vi "Run1TonWithoutWaveformDig.vi"() -> ()   [LabVIEW 2014]
doc: "Use this template to build a producer/consumer design pattern with events to produce queue items. Use this design pattern instead of the User Interface Event Handler pattern for user interfaces when you want to execute code asynchronously in response to an event without slowing the user interface responsiveness."
uses:
  <vilib>/addons/h5labview2/base/hid_t.ctl
  DatasetNames.ctl
  Program Files (x86)/CAEN/Comm/labview/CAENComm.lvlib
panel:
  out "Time Data (E-4 s)":T1
  in  "Monitoring Delay (ms)":u16=100 caption="Monitoring Delay (ms) (TDC, QDC, Dig, Time)"
  out "Duty Factor":dbl(graph)
  in  "?":T2(tab)
  out "TDC Histograms":u16[][](graph)
  out "QDC Histograms":u16[][](graph)
  out "Scaler Rates":T3(graph)
  in  "Scaler Delay (s)":sgl=10.0
  out "Time Histogram":u16[][](graph)
  in  "Max Hist Time (s)":sgl=0.25 format="%#_13g"
  in  "Time # Bins":i32=1000
  out "Temp Chart":dynamicdata(graph)
  out "Total Samples":sgl caption="Number of Samples Being Averaged"
  out "Mean":sgl
  in  "Temp Delay (s)":sgl=1.0
  in  "Max Samples":u32=600
  out "# elements in queue":i32
  out "Acquiring?":bool
  out "Scaler Data":u32[](array[numeric])
  out "Acquisition\nErrors":errorcluster
  in  "Clear Acquisition Errors":bool
  in  "QDC threshold":u16=1
  in  "Start Acquisition":bool
  out "# Events Written":i32
  in  "# Events to\nRecord":i32
  out "Analysis\nErrors":errorcluster
  in  "Calibrate Verniers":bool
  in  "Stop Acquisition":bool
  in  "Configure Output":bool
  in  "Calibrate Pedestals":bool
  in  "stop":bool
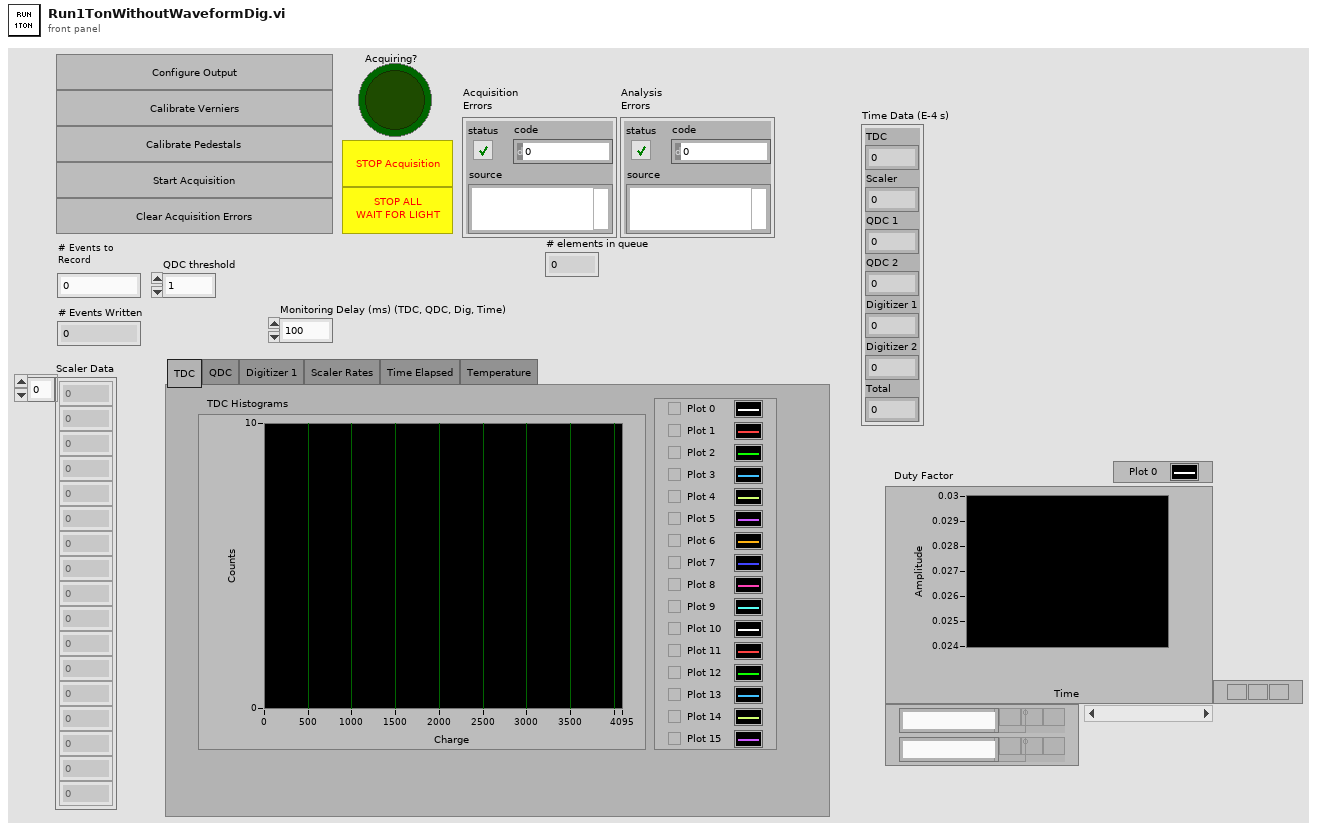
[diagram p1: front panel]
types:
  T1 = cluster{"TDC":u16, "Scaler":u16, "QDC 1":u16, "QDC 2":u16, "Digitizer 1":u16, "Digitizer 2":u16, "Total":u16}
  T2 = enum32{"TDC", "QDC", "Digitizer 1", "Scaler Rates", "Time Elapsed", "Temperature"}
  T3 = cluster{"[0]":dbl, "[1]":dbl, "[2]":dbl, "[3]":dbl}
  T4 = typedef "hid_t.ctl" = i32
  T5 = cluster{"State":enum16{"Startup", "Initialise", "Event OK", "Discard Event", "Exit", "Close"}, "Data":variant}
  T6 = typedef "DatasetNames.ctl" = enum16{"TDC", "Scaler", "QDC_1", "QDC_2", "Digitizer_1", "Digitizer_2", "Event_Time", "Event_Temp"}
  T7 = cluster{"TDC Data":u32[], "Scaler Data":u32[], "QDC 1 Data":u32[], "QDC 2 Data":u32[], "Event Start UNIX Time":dbl}
  T8 = enum16{"Startup", "Initialise", "Event OK", "Discard Event", "Exit", "Close"}
  T9 = cluster{"[0]":dbl, "[1]":dbl, "[2]":dbl, "[3]":dbl}[]
  T10 = cluster{"Channel":u8, "QDC Data":u16, "LowRange?":bool}[]
  T11 = cluster{"Data out[0]":u16, "Data out[1]":u16, "Data out[2]":u16, "Data out[3]":u16, "Data out[4]":u16, "Data out[5]":u16, "Data out[6]":u16}
  T12 = enum16{"Configure", "Initialise", "Run", "Close"}
  T13 = cluster{"TDC":u32, "Scaler":u32, "QDC 1":u32, "QDC 2":u32, "Digitizer 1":u32, "Digitizer 2":u32}
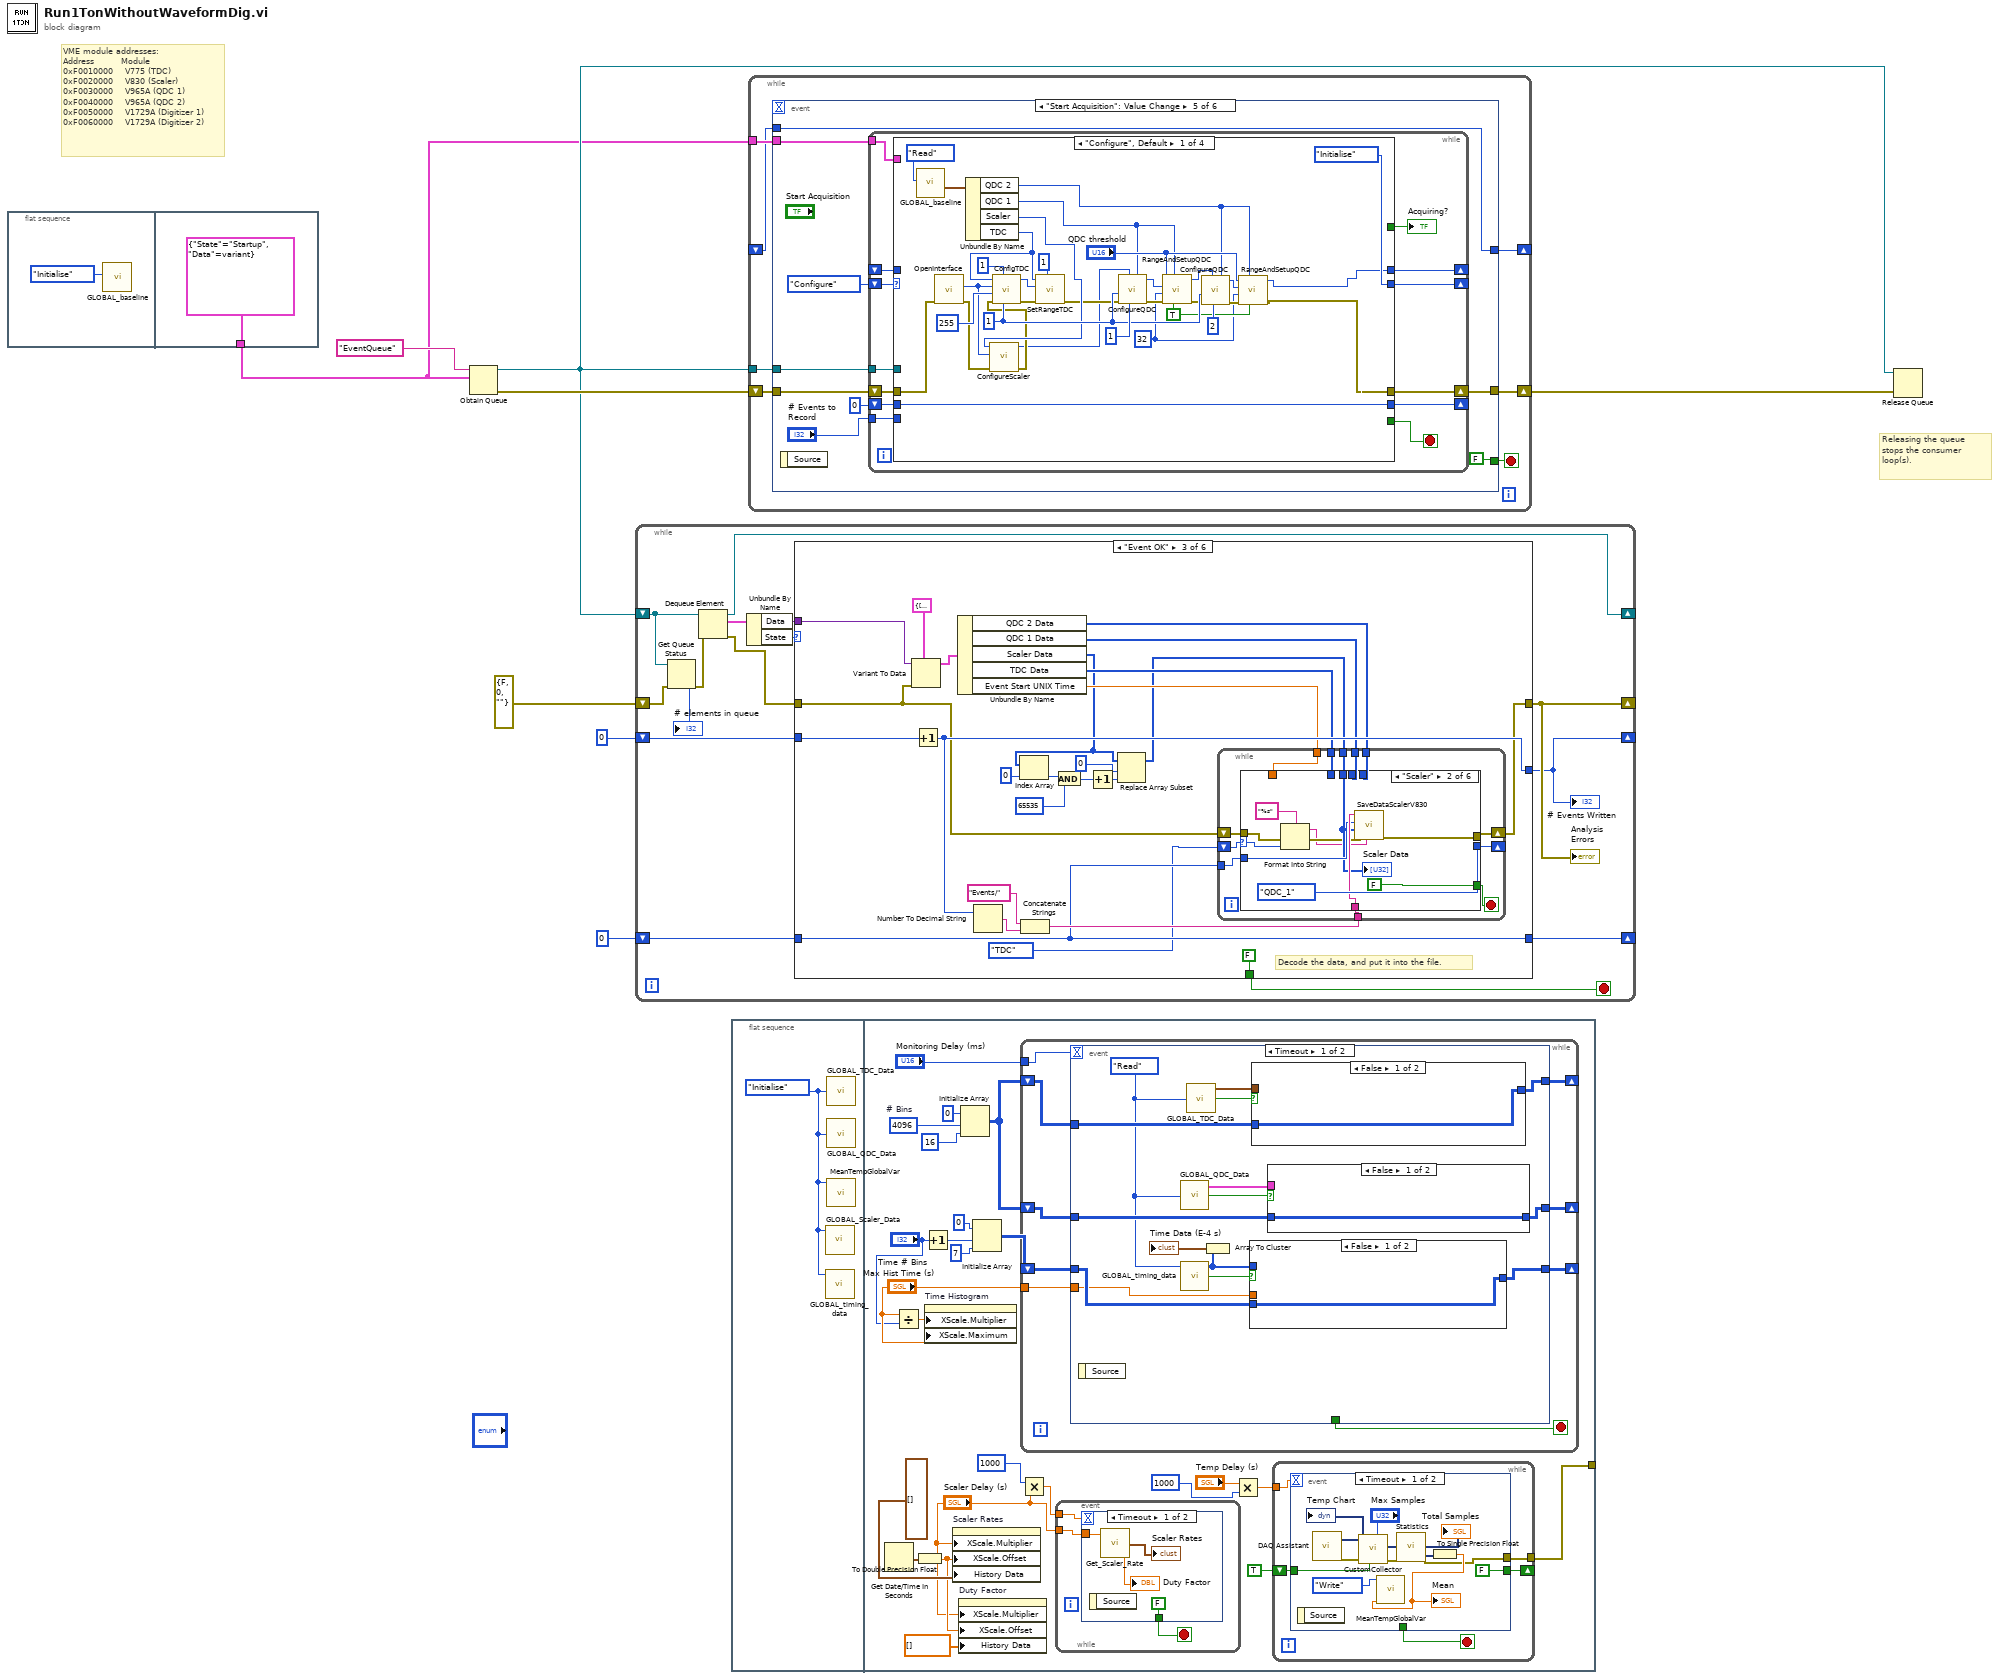
[diagram p0: block diagram]
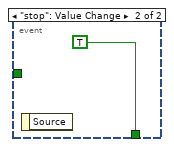
[diagram p2: hidden frame]
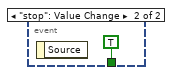
[diagram p3: hidden frame]
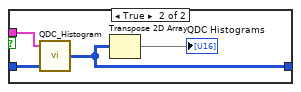
[diagram p4: hidden frame]
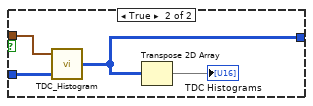
[diagram p5: hidden frame]
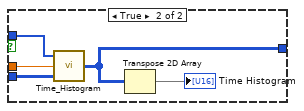
[diagram p6: hidden frame]
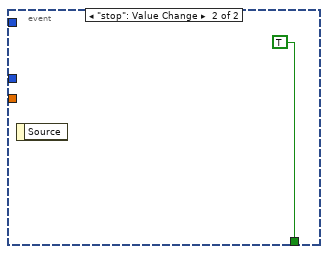
[diagram p7: hidden frame]
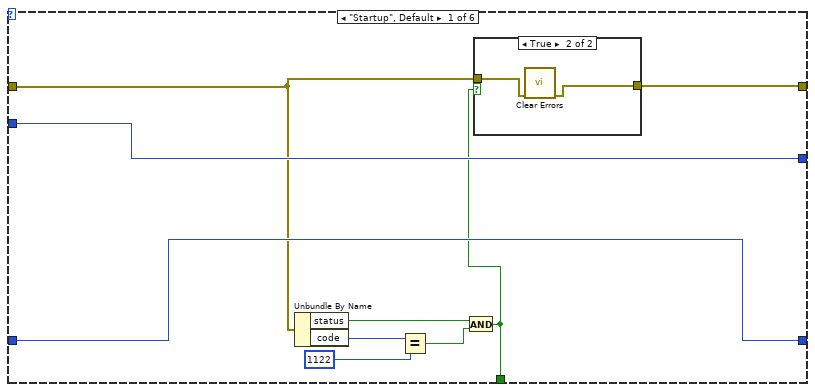
[diagram p8: hidden frame]
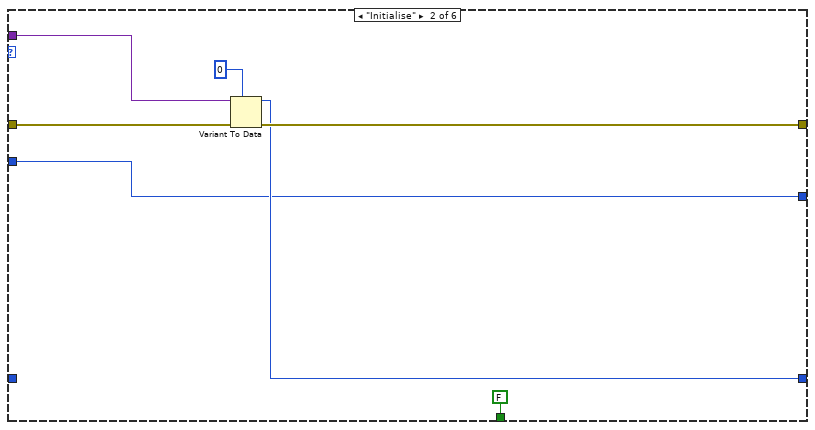
[diagram p10: hidden frame]
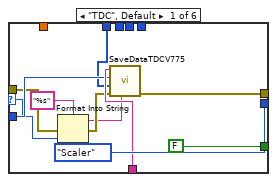
[diagram p11: hidden frame]
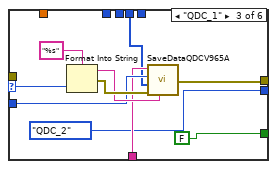
[diagram p12: hidden frame]
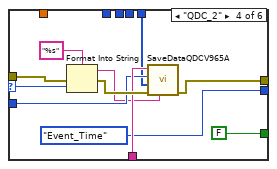
[diagram p13: hidden frame]
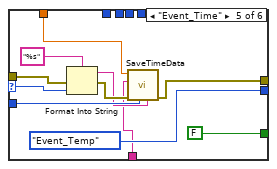
[diagram p14: hidden frame]
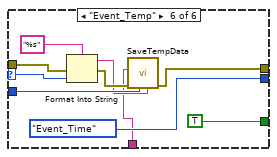
[diagram p15: hidden frame]
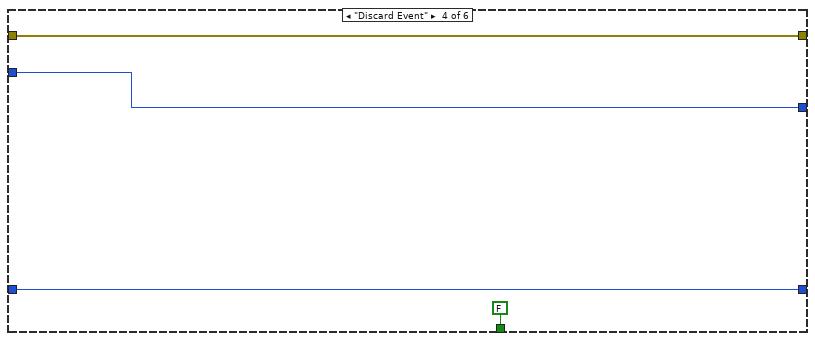
[diagram p16: hidden frame]
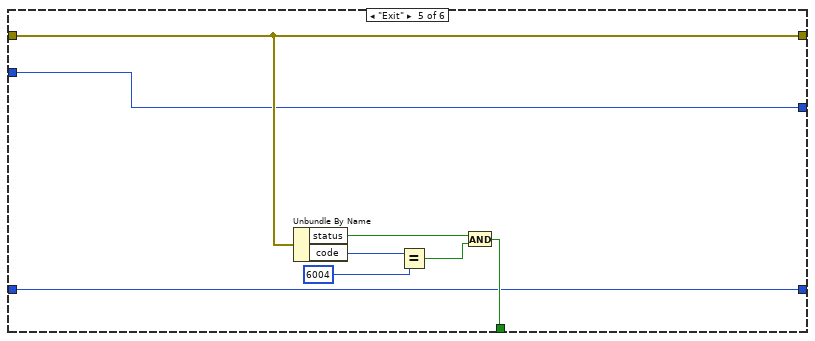
[diagram p17: hidden frame]
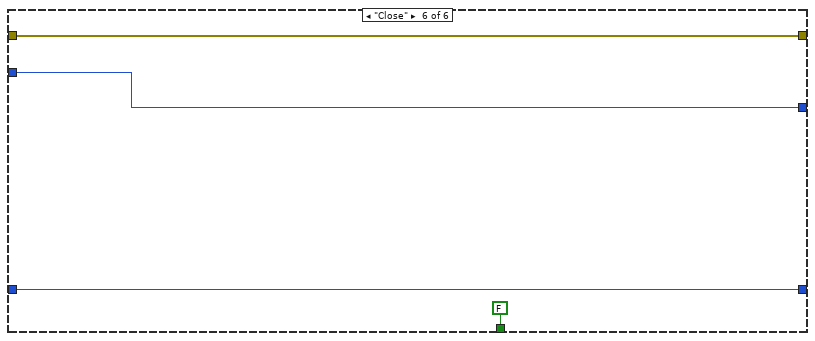
[diagram p18: hidden frame]
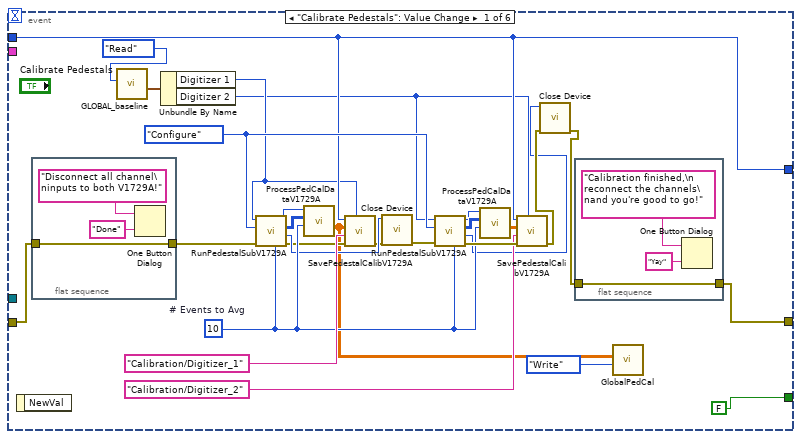
[diagram p19: hidden frame]
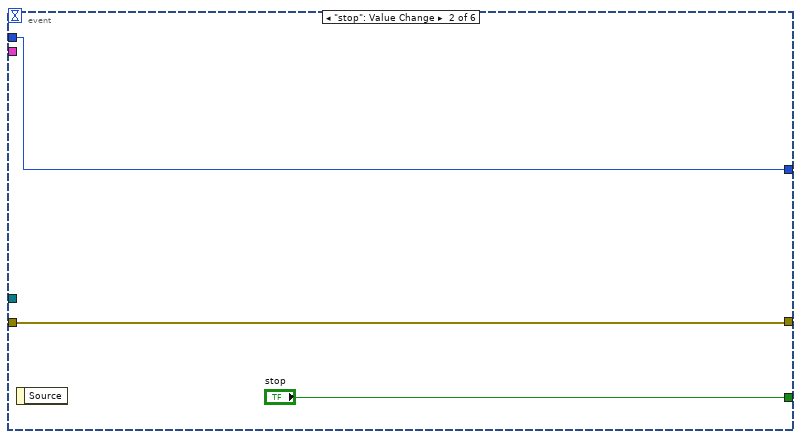
[diagram p20: hidden frame]
diagram:
  # "VME module addresses:\nAddress         Module\n0xF0010000    V775 (TDC)\n0xF0020000    V830 (Scaler)\n0xF0030000    V965A (QDC 1)\n0xF0040000    V965A (QDC 2)\n0xF0050000    V1729A (Digitizer 1)\n0xF0060000    V1729A (Digitizer 2)"
  # "Releasing the queue stops the consumer loop(s)."
  n1 = flat-sequence {
    tunnel: [T5 {"State"=enum."Startup", "Data"=variant}] -> w1
    frame #0 {
      n2 = call "GLOBAL_baseline.vi"("State"=enum16{"Initialise", "Write", "Read"}."Initialise") -> ()  [unwired: 10 in, 1 out]
    }
    frame #1 {
    }
  }
  n3 = Obtain Queue(name (unnamed)="EventQueue", element data type=w1) -> (queue out=w3:refnum<queue>, error out=w8:errorcluster)  [unwired: 3 in, 1 out]
  n4 = while {
    shift-right: [w16] -> _
    shift-left: errorcluster {"status"=FALSE, "code"=0, "source"=""} ("error out") -> [w14]
    shift-right: [w21] -> _
    shift-left: w3 -> [w12]
    shift-right: [w19] -> _
    shift-left: T4 0 ("File Handle") -> [w18]
    shift-right: [w15] -> _
    shift-left: 0 -> [w17]
    stop <- w20 stop-if-true
    n5 = Get Queue Status(queue=w12, error in (no error)=w14) -> (error out=w13:errorcluster, # elements in queue=→"# elements in queue":i32)  [unwired: 1 in, 6 out]
    n6 = Dequeue Element(queue=w12, error in (no error)=w13) -> (queue out=w21:refnum<queue>, element=w25:T5, error out=w22:errorcluster)  [unwired: 1 in, 1 out]
    n7 = Unbundle By Name(w25) -> ("Data"=w23:variant, "State"=w24:T8)
    n8 = case shown="\"Event OK\"" w24 {
      tunnel: w23 -> [_ w42 w68 _ _ _]
      tunnel: w22 -> [w28 w41 w57 w149 w152 w161]
      tunnel: [w26 w40 w55 w149 w152 w161] -> w16
      tunnel: [w27 FALSE FALSE FALSE w153 FALSE] -> w20
      tunnel: [w30 w39 w60 w147 w151 w159] -> w19
      tunnel: w18 -> [w30 _ w60 w147 w151 w159]
      tunnel: w17 -> [w29 w38 w67 w146 w150 w158]
      tunnel: [w29 w38 w66 w146 w150 w158] -> w15
      frame "Startup", Default {
        n9 = Unbundle By Name(w28) -> ("status"=w34:bool, "code"=w32:i32)
        n10 = Equal?(x=w32, y=1122) -> (x = y?=w33:bool)
        n11 = And(x=w34, y=w33) -> (x .and. y?=w27:bool)
        n12 = case shown="True" w27 {
          tunnel: w28 -> [w35 w37]
          tunnel: [w35 w36] -> w26
          frame False {
          }
          frame True {
            n13 = call <vilib>:"Clear Errors.vi"("error in (no error)"=w37) -> ("error out"=w36:errorcluster)  [unwired: 5 in, 1 out]
          }
        }
      }
      frame "Initialise" {
        n14 = Variant To Data(error in=w41, type=T4 0 ("File Handle"), Variant=w42) -> (data=w39:T4, error out=w40:errorcluster)
      }
      frame "Event OK" {
        # "Decode the data, and put it into the file."
        n15 = Variant To Data(error in=w57, type=T7 {"TDC Data"=[], "Scaler Data"=[], "QDC 1 Data"=[], "QDC 2 Data"=[], "Event Start UNIX Time"=0.0}, Variant=w68) -> (data=w62:T7)  [unwired: 1 out]
        n16 = Increment(x=w67) -> (x+1=w66:i32)
        n17 = Unbundle By Name(w62) -> ("QDC 2 Data"=w59:u32[], "QDC 1 Data"=w58:u32[], "Scaler Data"=w49:u32[], "TDC Data"=w56:u32[], "Event Start UNIX Time"=w53:dbl)
        n18 = Number To Decimal String(number=w66) -> (decimal integer string=w64:string)  [unwired: 1 in]
        n19 = Index Array(array=w49, index=0) -> (element=w51:u32)
        n20 = Concatenate Strings("Events/", w64) -> (w61:string)
        n21 = And(x=w51, y=u32 65535) -> (x .and. y?=w48:u32)
        n22 = Increment(x=w48) -> (x+1=w45:u32)
        n23 = Replace Array Subset(array=w49, new element=w45, index=0) -> (w46:u32[])
        n24 = while {
          tunnel: w61 -> [w81]
          tunnel: w60 -> [w80]
          tunnel: w59 -> [w78]
          tunnel: w58 -> [w77]
          shift-right: [w74] -> w55
          shift-left: w57 -> [w79]
          tunnel: w46 -> [w76]
          tunnel: w56 -> [w75]
          shift-right: [w73] -> _
          shift-left: DatasetNames."TDC" -> [w72]
          tunnel: w53 -> [w70]
          stop <- w71 stop-if-true
          n25 = case shown="\"Scaler\"" w72 {
            selector: w72 -> [w82 w96 w110 w123 w134 w144]
            tunnel: [w90 w101 w107 w116 w128 w138] -> w74
            tunnel: w80 -> [w88 w99 w109 w119 w129 w139]
            tunnel: w81 -> [w89 w100 w108 w120 w126 w136]
            tunnel: w79 -> [w85 w95 _ w122 w131 w141]
            tunnel: w78 -> [_ _ _ w118 _ _]
            tunnel: w77 -> [_ _ w106 _ _ _]
            tunnel: [DatasetNames."Scaler" DatasetNames."QDC_1" DatasetNames."QDC_2" DatasetNames."Event_Time" DatasetNames."Event_Temp" DatasetNames."Event_Time"] -> w73
            tunnel: [FALSE FALSE FALSE FALSE FALSE TRUE] -> w71
            tunnel: w76 -> [_ w98 _ _ _ _]
            tunnel: w75 -> [w87 _ _ _ _ _]
            tunnel: w70 -> [_ _ _ _ w125 _]
            frame "TDC", Default {
              n26 = Format Into String(format string="%s", error in=w85, w82) -> (resulting string=w83:string, error out=w84:errorcluster)  [unwired: 1 in]
              n27 = call "SaveDataTDCV775.vi"("Module"=w83, "error in (no error)"=w84, "Buff"=w87, "File Handle"=w88, "String"=w89) -> ("error out"=w90:errorcluster)  [unwired: 5 in, 1 out]
            }
            frame "Scaler" {
              n28 = Format Into String(format string="%s", error in=w95, w96) -> (resulting string=w93:string, error out=w94:errorcluster)  [unwired: 1 in]
              n29 = call "SaveDataScalerV830.vi"("Module"=w93, "error in (no error)"=w94, "Buff"=w98, "File Handle"=w99, "Group Name"=w100) -> ("error out"=w101:errorcluster)  [unwired: 6 in]
              "Scaler Data" <- w98
            }
            frame "QDC_1" {
              n30 = Format Into String(format string="%s", w110) -> (resulting string=w111:string, error out=w112:errorcluster)  [unwired: 2 in]
              n31 = call "SaveDataQDCV965A.vi"("Module"=w111, "error in (no error)"=w112, "Buff"=w106, "File Handle"=w109, "String"=w108) -> ("error out"=w107:errorcluster)  [unwired: 5 in, 1 out]
            }
            frame "QDC_2" {
              n32 = Format Into String(format string="%s", error in=w122, w123) -> (resulting string=w117:string, error out=w121:errorcluster)  [unwired: 1 in]
              n33 = call "SaveDataQDCV965A.vi"("Module"=w117, "error in (no error)"=w121, "Buff"=w118, "File Handle"=w119, "String"=w120) -> ("error out"=w116:errorcluster)  [unwired: 5 in, 1 out]
            }
            frame "Event_Time" {
              n34 = Format Into String(format string="%s", error in=w131, w134) -> (resulting string=w127:string, error out=w130:errorcluster)  [unwired: 1 in]
              n35 = call "SaveTimeData.vi"("Module"=w127, "File Handle"=w129, "error in (no error)"=w130, "String"=w126, "Event Start UNIX Time"=w125) -> ("error out"=w128:errorcluster)  [unwired: 5 in, 1 out]
            }
            frame "Event_Temp" {
              n36 = Format Into String(format string="%s", error in=w141, w144) -> (resulting string=w137:string, error out=w140:errorcluster)  [unwired: 1 in]
              n37 = call "SaveTempData.vi"("Module"=w137, "File Handle"=w139, "error in (no error)"=w140, "String"=w136) -> ("error out"=w138:errorcluster)  [unwired: 6 in, 1 out]
            }
          }
        }
      }
      frame "Discard Event" {
      }
      frame "Exit" {
        n38 = Unbundle By Name(w152) -> ("status"=w157:bool, "code"=w155:i32)
        n39 = Equal?(x=w155, y=6004) -> (x = y?=w156:bool)
        n40 = And(x=w157, y=w156) -> (x .and. y?=w153:bool)
      }
      frame "Close" {
      }
    }
    "Analysis\nErrors" <- w16
    "# Events Written" <- w15
  }
  n41 = flat-sequence {
    tunnel: [w163] -> _
    frame #0 {
      w162 = enum16{"Initialise", "Write", "Read"}."Initialise" ("State")
      n42 = call "GLOBAL_Scaler_Data.vi"("State"=w162) -> ()  [unwired: 3 in, 2 out]
      n43 = call "GLOBAL_timing_data.vi"("State"=w162) -> ()  [unwired: 3 in, 2 out]
      n44 = call "GLOBAL_TDC_Data.vi"("State"=w162) -> ()  [unwired: 3 in, 2 out]
      n45 = call "GLOBAL_QDC_Data.vi"("State"=w162) -> ()  [unwired: 3 in, 2 out]
      n46 = call "MeanTempGlobalVar.vi"("State"=w162) -> ()  [unwired: 10 in, 1 out]
    }
    frame #1 {
      w185 = u16 4096  # # Bins
      n47 = Get Date/Time In Seconds() -> (seconds since 1Jan1904=w182:timestamp)
      n48 = Divide(x="Max Hist Time (s)", y="Time # Bins") -> (x/y=w177:sgl)
      n49 = To Double Precision Float(number=w182) -> (double precision float=w173:dbl)
      n50 = Increment(x="Time # Bins") -> (x+1=w175:i32)
      n51 = property on="Time Histogram" class="WFGraph (strict)"("XScale.Multiplier"=w177, "XScale.Maximum"="Max Hist Time (s)") -> ()  [unwired: 2 in, 2 out]
      n52 = property on="Scaler Rates" class="WFChart (strict)"("XScale.Multiplier"="Scaler Delay (s)", "XScale.Offset"=w173, "History Data"=T9 []) -> ()  [unwired: 2 in, 2 out]
      n53 = property on="Duty Factor" class="WFChart (strict)"("XScale.Multiplier"="Scaler Delay (s)", "XScale.Offset"=w173, "History Data"=dbl[] []) -> ()  [unwired: 2 in, 2 out]
      n54 = Initialize Array(u16 0 ("element"), w185, 16 ("dimension size")) -> (w183:u16[][])
      n55 = Initialize Array(u16 0 ("element"), w175, 7 ("dimension size")) -> (w178:u16[][])
      n56 = Multiply(x=u32 1000 ("y"), y="Scaler Delay (s)") -> (x*y=w168:sgl)
      n57 = while {
        shift-right: [w215] -> _
        shift-left: w183 -> [w220]
        shift-right: [w217] -> _
        shift-left: w183 -> [w219]
        shift-right: [w216] -> _
        shift-left: w178 -> [w218]
        tunnel: "Max Hist Time (s)" -> [w221]
        tunnel: "Monitoring Delay (ms)" -> [w213]
        stop <- w214 stop-if-true
        n58 = event shown="[0] Timeout" {
          selector: _ -> [_ _]
          dyn-events: _ -> [_ _]
          timeout: w213 -> [_ _]
          tunnel: w221 -> [w228 _]
          tunnel: w220 -> [w231 _]
          tunnel: w219 -> [w230 _]
          tunnel: w218 -> [w229 _]
          tunnel: [w227 _] -> w217
          tunnel: [w226 _] -> w216
          tunnel: [w225 _] -> w215
          tunnel: [_ TRUE] -> w214
          event Timeout {
            w222 = enum16{"Initialise", "Write", "Read"}."Read" ("State")
            n59 = event-data() -> ()  [unwired: 1 in, 1 out]
            n60 = call "GLOBAL_QDC_Data.vi"("State"=w222) -> ("Valid Read?"=w234:bool, "Data Out"=w233:T10)  [unwired: 3 in]
            n61 = call "GLOBAL_timing_data.vi"("State"=w222) -> ("Valid Read?"=w232:bool, "Data out"=w224:u16[])  [unwired: 3 in]
            n62 = call "GLOBAL_TDC_Data.vi"("State"=w222) -> ("Valid Read?"=w236:bool, "Data Out"=w235:cluster{"Channel":u8, "TDC Data":u16}[])  [unwired: 3 in]
            n63 = Array To Cluster(array=w224) -> (cluster=→"Time Data (E-4 s)":T11)
            n64 = case shown="False" w232 {
              tunnel: w224 -> [_ w252]
              tunnel: [w247 w250] -> w226
              tunnel: w229 -> [w247 w249]
              tunnel: w228 -> [_ w248]
              frame False {
              }
              frame True {
                n65 = call "Time_Histogram.vi"("Hist array in"=w249, "Max (s)"=w248, "Data in"=w252) -> ("Hist array out"=w250:u16[][])  [unwired: 2 in]
                n66 = Transpose 2D Array(2D array=w250) -> (transposed array=→"Time Histogram":u16[][])
              }
            }
            n67 = case shown="False" w236 {
              tunnel: w235 -> [_ w246]
              tunnel: [w242 w244] -> w225
              tunnel: w231 -> [w242 w243]
              frame False {
              }
              frame True {
                n68 = call "TDC_Histogram.vi"("Hist array in"=w243, "Data In"=w246) -> ("Hist array out"=w244:u16[][])  [unwired: 3 in]
                n69 = Transpose 2D Array(2D array=w244) -> (transposed array=→"TDC Histograms":u16[][])
              }
            }
            n70 = case shown="False" w234 {
              tunnel: w233 -> [_ w241]
              tunnel: [w237 w239] -> w227
              tunnel: w230 -> [w237 w238]
              frame False {
              }
              frame True {
                n71 = call "QDC_Histogram.vi"("Hist array in"=w238, "Data In"=w241) -> ("Hist array out"=w239:u16[][])  [unwired: 3 in]
                n72 = Transpose 2D Array(2D array=w239) -> (transposed array=→"QDC Histograms":u16[][])
              }
            }
          }
          event "stop": Value Change {
            n73 = event-data() -> ()  [unwired: 1 in, 1 out]
          }
        }
      }
      n74 = while {
        tunnel: "Scaler Delay (s)" -> [w206]
        tunnel: w168 -> [w205]
        stop <- w207 stop-if-true
        n75 = event shown="[0] Timeout" {
          selector: _ -> [_ _]
          dyn-events: _ -> [_ _]
          timeout: w205 -> [_ _]
          tunnel: w206 -> [w211 _]
          tunnel: [FALSE TRUE] -> w207
          event Timeout {
            n76 = event-data() -> ()  [unwired: 1 in, 1 out]
            n77 = call "Get_Scaler_Rate.vi"("Delay Time (s)"=w211) -> ("Duty Factor"=→"Duty Factor":dbl, "Cluster out"=→"Scaler Rates":T3)  [unwired: 3 in]
          }
          event "stop": Value Change {
            n78 = event-data() -> ()  [unwired: 1 in, 1 out]
          }
        }
      }
      n79 = Multiply(x="Temp Delay (s)", y=u16 1000) -> (x*y=w170:sgl)
      n80 = while {
        shift-right: [w191] -> _
        shift-left: TRUE -> [w189]
        tunnel: w170 -> [w188]
        tunnel: [w187] -> w163
        stop <- w190 stop-if-true
        n81 = event shown="[0] Timeout" {
          selector: _ -> [_ _]
          dyn-events: _ -> [_ _]
          timeout: w188 -> [_ _]
          tunnel: [FALSE _] -> w191
          tunnel: w189 -> [w192 _]
          tunnel: [_ TRUE] -> w190
          tunnel: [w193 _] -> w187
          event Timeout {
            n82 = event-data() -> ()  [unwired: 1 in, 1 out]
            n83 = call "DAQ Assistant"() -> ("data"=w196:dynamicdata, "error out"=w202:errorcluster)  [unwired: 17 in, 1 out]
            "Temp Chart" <- w196
            n84 = call "CustomCollector.vi"("Reset"=w192, "error in (no error)"=w202, "Size"="Max Samples", "Signals"=w196) -> ("error out"=w201:errorcluster, "Collected Signals"=w203:dynamicdata)  [unwired: 6 in]
            n85 = call "Statistics"("Signals"=w203, "error in (no error)"=w201) -> ("Total Samples"=→"Total Samples":dynamicdata, "Arithmetic Mean"=w199:dynamicdata, "error out"=w193:errorcluster)  [unwired: 23 in]
            n86 = To Single Precision Float(number=w199) -> (single precision float=w198:sgl)
            "Mean" <- w198
            n87 = call "MeanTempGlobalVar.vi"("Temp In"=w198, "State"=enum16{"Initialise", "Write", "Read"}."Write") -> ()  [unwired: 9 in, 1 out]
          }
          event "stop": Value Change {
            n88 = event-data() -> ()  [unwired: 1 in, 1 out]
          }
        }
      }
    }
  }
  n89 = while {
    shift-right: [w258] -> w5
    shift-left: w8 -> [w259]
    tunnel: w3 -> [w260]
    tunnel: w1 -> [w256]
    shift-right: [w255] -> _
    shift-left: _ -> [w254]
    stop <- w257 stop-if-true
    n90 = event shown="[4] \"Start Acquisition\": Value Change" {
      selector: _ -> [_ _ _ _ _ _]
      dyn-events: _ -> [_ _ _ _ _ _]
      timeout: _ -> [_ _ _ _ _ _]
      tunnel: w260 -> [_ _ _ w302 w314 _]
      tunnel: w259 -> [w264 w297 _ w303 w316 w428]
      tunnel: [w283 w297 _ w306 _ w427] -> w258
      tunnel: [FALSE ("stop") "stop" FALSE ("stop") FALSE ("stop") FALSE ("stop") _] -> w257
      tunnel: w256 -> [_ _ _ w307 w315 _]
      tunnel: [w282 w296 w298 w300 w311 _] -> w255
      tunnel: w254 -> [w282 w296 w298 _ w311 _]
      event "Calibrate Pedestals": Value Change {
        w286 = T12."Configure"
        w277 = 10  # # Events to Avg
        n91 = event-data() -> ()  [unwired: 1 in, 1 out]
        n92 = flat-sequence {
          tunnel: w264 -> [w294]
          tunnel: [w294] -> w274
          frame #0 {
            n93 = One Button Dialog(message="Disconnect all channel\ninputs to both V1729A!", button name ("OK")="Done") -> ()  [unwired: 1 out]
          }
        }
        n94 = call "GLOBAL_baseline.vi"("State"=enum16{"Initialise", "Write", "Read"}."Read") -> ("Addresses Out"=w280:T13)  [unwired: 10 in]
        n95 = Unbundle By Name(w280) -> ("Digitizer 1"=w273:u32, "Digitizer 2"=w270:u32)
        n96 = call "RunPedestalSubV1729A.vi"("# Events to Avg"=w277, "error in (no error)"=w274, "Init State"=w286, "VME Base Address in"=w273) -> ("error out"=w267:errorcluster, "handle out"=w272:i32, "Data Out"=w287:u32[][], "Offset"=w266:i16)  [unwired: 4 in]
        n97 = call "ProcessPedCalDataV1729A.vi"("# Events to Avg"=w277, "Data In"=w287, "Offset"=w266) -> ("Channel Data"=w261:dbl[][])  [unwired: 8 in]
        n98 = call "SavePedestalCalibV1729A.vi"("Address"=w273, "error in (no error)"=w267, "Group Name"="Calibration/Digitizer_1", "Data In"=w261, "File Handle"=w282) -> ("error out"=w269:errorcluster)  [unwired: 6 in]
        n99 = call "Close Device.vi"("error in (no error)"=w269, "handle"=w272) -> ("error out"=w268:errorcluster)  [unwired: 9 in]
        n100 = call "RunPedestalSubV1729A.vi"("# Events to Avg"=w277, "error in (no error)"=w268, "Init State"=w286, "VME Base Address in"=w270) -> ("error out"=w284:errorcluster, "handle out"=w271:i32, "Data Out"=w285:u32[][], "Offset"=w265:i16)  [unwired: 4 in]
        n101 = call "ProcessPedCalDataV1729A.vi"("# Events to Avg"=w277, "Data In"=w285, "Offset"=w265) -> ("Channel Data"=w262:dbl[][])  [unwired: 8 in]
        n102 = call "SavePedestalCalibV1729A.vi"("Address"=w270, "error in (no error)"=w284, "Group Name"="Calibration/Digitizer_2", "Data In"=w262, "File Handle"=w282) -> ("error out"=w276:errorcluster)  [unwired: 6 in]
        n103 = call "Close Device.vi"("error in (no error)"=w276, "handle"=w271) -> ("error out"=w275:errorcluster)  [unwired: 9 in]
        n104 = flat-sequence {
          tunnel: w275 -> [w289]
          tunnel: [w289] -> w283
          frame #0 {
            n105 = One Button Dialog(message="Calibration finished,\n reconnect the channels\nand you're good to go!", button name ("OK")="Yay") -> ()  [unwired: 1 out]
          }
        }
        n106 = call "GlobalPedCal.vi"("State"=enum16{"Initialise", "Write", "Read"}."Write", "Data In"=w261) -> ()  [unwired: 9 in, 1 out]
      }
      event "stop": Value Change {
        n107 = event-data() -> ()  [unwired: 1 in, 1 out]
      }
      event "Calibrate Verniers": Value Change {
        # "This needs to be implemented if we want better timing resolution on the digitizers (apparently ~70 ps)\n- The user will need to feed in a sawtooth waveform.\n- This calibration will determine MINVER and MAXVER for each digitizer (see V1729A manual)\n- The MINVER and MAXVER correction can be applied offline (or online if we can spare the delay)."
        n108 = event-data() -> ()  [unwired: 1 in, 1 out]
      }
      event "Configure Output": Value Change {
        w308 = T8."Initialise"  # State
        n109 = event-data() -> ()  [unwired: 1 in, 1 out]
        n110 = call "CreateHDF5NoDig.vi"() -> ("error out"=w305:errorcluster, "File Handle"=w300:T4)  [unwired: 10 in]
        n111 = To Variant(anything=w300) -> (Variant=w309:variant)
        n112 = Bundle By Name(cluster=w307, "State"=w308, "Data"=w309) -> (w301:T5)
        n113 = Enqueue Element(queue=w302, element=w301, error in (no error)=w303) -> (error out=w304:errorcluster)  [unwired: 1 in, 2 out]
        n114 = Merge Errors(w305, w304) -> (w306:errorcluster)
      }
      event "Start Acquisition": Value Change {
        n115 = event-data() -> ()  [unwired: 1 in, 1 out]
        n116 = while {
          shift-right: [w326] -> _
          shift-left: T12."Configure" -> [w331]
          shift-right: [w329] -> _
          shift-left: w316 -> [w330]
          shift-right: [w328] -> _
          shift-left: _ -> [w327]
          tunnel: w315 -> [w325]
          tunnel: w314 -> [w324]
          tunnel: "# Events to\nRecord" -> [w322]
          shift-right: [w320] -> _
          shift-left: 0 -> [w323]
          stop <- w321 stop-if-true
          n117 = case shown="\"Configure\", Default" w331 {
            tunnel: w330 -> [w364 w380 w405 w417]
            tunnel: [w332 w381 w399 w423] -> w329
            tunnel: [w333 w371 w387 w415] -> w328
            tunnel: w327 -> [_ w379 w387 w415]
            tunnel: [T12."Initialise" T12."Run" w396 T12."Close"] -> w326
            tunnel: w325 -> [_ _ w402 w419]
            tunnel: w324 -> [_ _ w401 w422]
            tunnel: w323 -> [w362 w382 w395 w424]
            tunnel: w322 -> [_ _ w394 _]
            tunnel: [_ _ _ TRUE] -> w321
            tunnel: [w362 w382 w392 w424] -> w320
            tunnel: [_ _ TRUE _] -> w319
            frame "Configure", Default {
              w347 = u16 32 ("High range threshold")
              w348 = TRUE ("Count only accepted trigs?\n(else all trigs)")
              w355 = u16 1 ("# Evts to Acquire")
              n118 = call "GLOBAL_baseline.vi"("State"=enum16{"Initialise", "Write", "Read"}."Read") -> ("Addresses Out"=w343:T13)  [unwired: 10 in]
              n119 = call "OpenInterface.vi"("error in (no error)"=w364) -> ("error out"=w339:errorcluster, "handle"=w338:i32)  [unwired: 8 in, 1 out]
              n120 = Unbundle By Name(w343) -> ("QDC 2"=w340:u32, "QDC 1"=w341:u32, "Scaler"=w337:u32, "TDC"=w342:u32)
              n121 = call "ConfigureScaler.vi"("error in (no error)"=w339, "handle"=w338, "VME Base Address"=w337) -> ("error out"=w336:errorcluster, "handle out"=w334:i32)  [unwired: 6 in, 1 out]
              n122 = call "ConfigTDC.vi"("# Evts to Acquire"=w355, "Interrupt Level"=u16 1, "error in (no error)"=w336, "FSR setting"=u16 255, "handle"=w338, "VME Base Address"=w342) -> ("error out"=w359:errorcluster, "handle out"=w358:i32)  [unwired: 4 in]
              n123 = call "SetRangeTDC.vi"("Low Range threshold"=u16 1, "error in (no error)"=w359, "handle"=w358, "VME module Base Address"=w342) -> ("error out"=w335:errorcluster)  [unwired: 5 in, 2 out]
              n124 = call "ConfigureQDC.vi"("VME module Base Address"=w341, "IRQ Lvl"=u16 1, "handle"=w334, "error in (no error)"=w335, "# of events before transfer (max 32)"=w355) -> ("error out"=w353:errorcluster, "handle out"=w352:i32)  [unwired: 5 in]
              n125 = call "RangeAndSetupQDC.vi"("Count only accepted trigs?\n(else all trigs)"=w348, "VME module Base Address"=w341, "error in (no error)"=w353, "High range threshold"=w347, "handle in"=w352, "Low Range threshold"="QDC threshold") -> ("error out"=w351:errorcluster, "handle out"=w350:i32)  [unwired: 4 in]
              n126 = call "ConfigureQDC.vi"("VME module Base Address"=w340, "IRQ Lvl"=u16 2, "handle"=w350, "error in (no error)"=w351, "# of events before transfer (max 32)"=w355) -> ("error out"=w349:errorcluster, "handle out"=w345:i32)  [unwired: 5 in]
              n127 = call "RangeAndSetupQDC.vi"("Count only accepted trigs?\n(else all trigs)"=w348, "VME module Base Address"=w340, "error in (no error)"=w349, "High range threshold"=w347, "handle in"=w345, "Low Range threshold"="QDC threshold") -> ("error out"=w332:errorcluster, "handle out"=w333:i32)  [unwired: 4 in]
            }
            frame "Initialise" {
              n128 = call "GLOBAL_baseline.vi"("State"=enum16{"Initialise", "Write", "Read"}."Read") -> ("Addresses Out"=w369:T13)  [unwired: 10 in]
              n129 = Unbundle By Name(w369) -> ("QDC 2"=w365:u32, "QDC 1"=w366:u32, "Scaler"=w367:u32, "TDC"=w368:u32)
              n130 = call "ClearEventsTDC.vi"("error in (no error)"=w380, "handle"=w379, "VME module Base Address"=w368) -> ("error out"=w378:errorcluster, "handle out"=w377:i32)  [unwired: 6 in, 1 out]
              n131 = call "ClearEventsV830.vi"("error in (no error)"=w378, "handle in"=w377, "VME Base Address"=w367) -> ("error out"=w376:errorcluster, "handle out"=w375:i32)  [unwired: 7 in]
              n132 = call "ClearEventsQDC.vi"("error in (no error)"=w376, "handle"=w375, "VME module Base Address"=w366) -> ("error out"=w374:errorcluster, "handle out"=w373:i32)  [unwired: 6 in, 1 out]
              n133 = call "ClearEventsQDC.vi"("error in (no error)"=w374, "handle"=w373, "VME module Base Address"=w365) -> ("error out"=w372:errorcluster, "handle out"=w371:i32)  [unwired: 6 in, 1 out]
              n134 = call "IRQ Enable.vi"("error in (no error)"=w372, "handle"=w371) -> ("error out"=w381:errorcluster)  [unwired: 9 in]
            }
            frame "Run" {
              # "Acquire"
              n135 = call <vilib>:"Clear Errors.vi"("error in (no error)"=w405, "specific error code to clear (0: all)"=-7) -> ("error out"=w384:errorcluster)  [unwired: 4 in, 1 out]
              "Acquisition\nErrors" <- w384
              n136 = Increment(x=w395) -> (x+1=w392:i32)
              n137 = Greater Or Equal?(x=w392, y=w394) -> (x >= y?=w393:bool)
              n138 = while {
                tunnel: w384 -> [w412]
                tunnel: [w411] -> w385
                tunnel: w387 -> [w410]
                shift-right: [w409] -> _
                shift-left: u8 0 ("Mask") -> [w407]
                stop <- w406 stop-if-true
                n139 = Equal?(x=w407, y=u8 7) -> (x = y?=w406:bool)
                n140 = call "VMEIRQ Check.vi"("error in (no error)"=w412, "VMEhandle"=w410) -> ("error out"=w411:errorcluster, "Mask"=w409:u8)  [unwired: 8 in]
              }
              n141 = Or(x=w393, y="Stop Acquisition") -> (x .or. y?=w397:bool)
              n142 = call "GetAllDataNoDig.vi"("error in (no error)"=w385, "handle in"=w387) -> ("error out"=w386:errorcluster, "Data out"=w390:T7)  [unwired: 7 in, 1 out]
              n143 = case shown="False" w397 {
                tunnel: [T12."Run" T12."Close"] -> w396
                frame False {
                }
                frame True {
                }
              }
              n144 = To Variant(anything=w390) -> (Variant=w404:variant)
              n145 = Bundle By Name(cluster=w402, "State"=T8."Event OK", "Data"=w404) -> (w400:T5)
              n146 = Enqueue Element(queue=w401, element=w400, error in (no error)=w386) -> (error out=w399:errorcluster)  [unwired: 1 in, 2 out]
            }
            frame "Close" {
              n147 = call "Close Device.vi"("error in (no error)"=w417, "handle"=w415) -> ("error out"=w416:errorcluster)  [unwired: 9 in]
              n148 = Bundle By Name(cluster=w419, "State"=T8."Close", "Data"=variant) -> (w418:T5)
              n149 = Enqueue Element(queue=w422, element=w418, error in (no error)=w416) -> (error out=w423:errorcluster)  [unwired: 1 in, 2 out]
            }
          }
          "Acquiring?" <- w319
        }
      }
      event "Clear Acquisition Errors": Value Change {
        n150 = event-data() -> ()  [unwired: 1 in, 2 out]
        n151 = call <vilib>:"Clear Errors.vi"("error in (no error)"=w428) -> ("error out"=w427:errorcluster)  [unwired: 5 in, 1 out]
      }
    }
  }
  n152 = Release Queue(queue=w3, error in (no error)=w5) -> ()  [unwired: 1 in, 3 out]
